vi "Set_ADODB._Recordset.vi"(8 "error in (no error)":errorcluster caption="错误输入（无错误）", 10 "ADODB._Recordset":refnum<k7>, 11 "Database Recordset输入":refnum<class "Database Recordset.lvclass">) -> (0 "error out":errorcluster caption="错误输出", 3 "Database Recordset输出":refnum<class "Database Recordset.lvclass">)   [LabVIEW 2011, in "Database Recordset.lvclass"]
uses:
  Database Recordset.lvclass
  Database Recordset.lvclass/Database Recordset.ctl
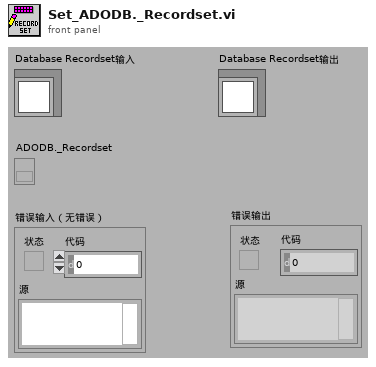
[diagram p1: front panel]
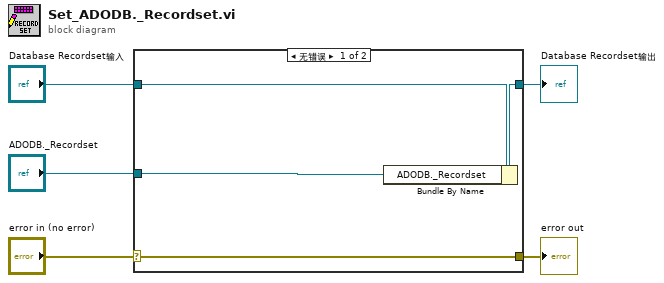
[diagram p0: block diagram]
diagram:
  n1 = case shown="无错误" "error in (no error)" {
    selector: "error in (no error)" -> [w9 w10]
    tunnel: [w9 w10] -> w4
    tunnel: [w7 w11] -> w2
    tunnel: "Database Recordset输入" -> [w8 w11]
    tunnel: "ADODB._Recordset" -> [w6 _]
    frame No Error {
      n2 = Bundle By Name(cluster=w8, "ADODB._Recordset"=w6) -> (w7:refnum<class "Database Recordset.lvclass">)
    }
    frame Error {
    }
  }
  "error out" <- w4
  "Database Recordset输出" <- w2
